vi "Delete last element.vi"(8 "error in":errorcluster, 11 "Path in":string) -> (0 "error out":errorcluster, 2 "Path Array Out":string[](array[string]), 3 "Element Array Out":string[](array[string]))   [LabVIEW 2015]
uses:
  <vilib>/regexp/Match Regular Expression.xnode
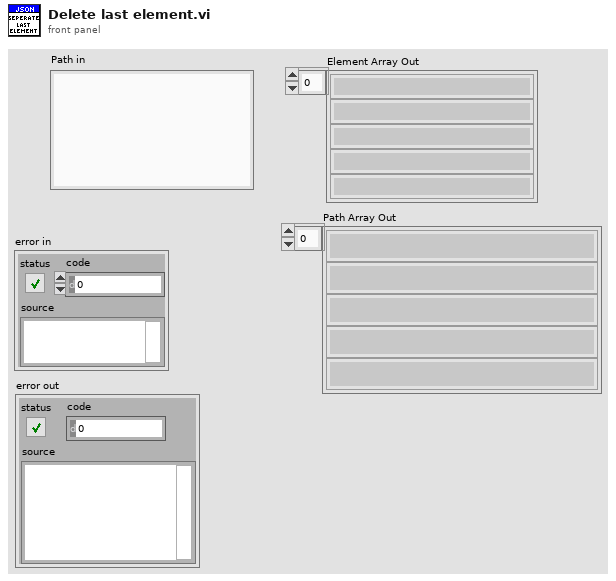
[diagram p1: front panel]
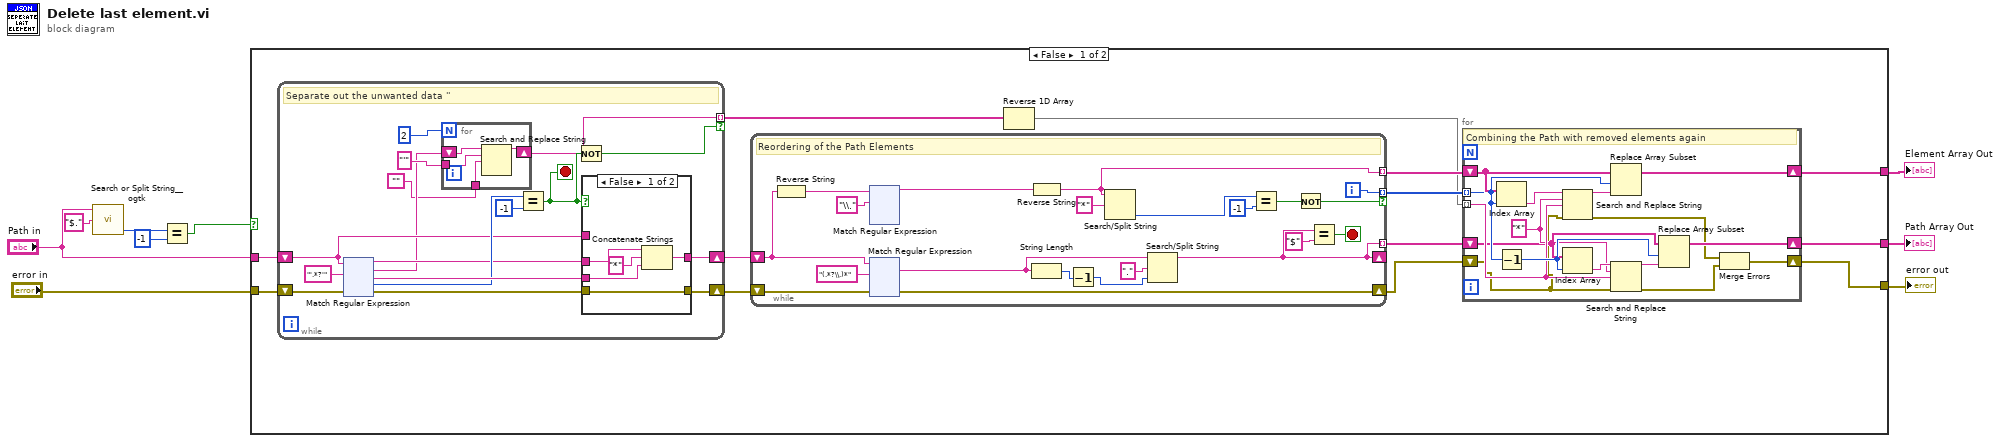
[diagram p0: block diagram]
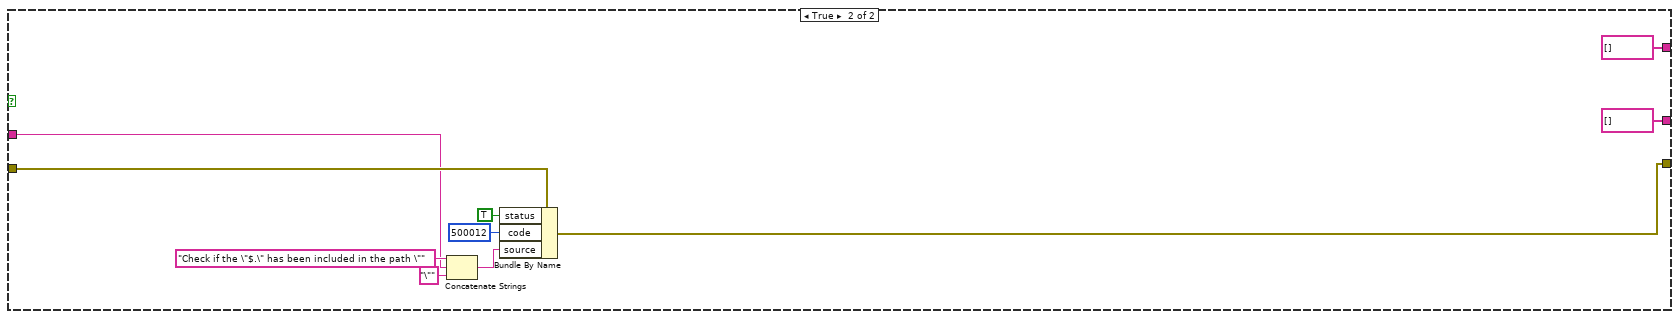
[diagram p3: hidden frame]
diagram:
  n1 = call <userlib>:"Search or Split String__ogtk.vi"("search string/char (-)"="$.", "string"="Path in") -> ("offset after match"=w3:i32)  [unwired: 1 in, 2 out]
  n2 = Equal?(x=w3, y=-1) -> (x = y?=w1:bool)
  n3 = case shown="False" w1 {
    tunnel: [w18 string[] []] -> w9
    tunnel: [w17 string[] []] -> w8
    tunnel: "error in" -> [w16 w439]
    tunnel: [w13 w432] -> w6
    tunnel: "Path in" -> [w10 w435]
    frame False {
      n4 = while {
        shift-right: [w302] -> w22
        shift-left: w10 -> [w298]
        tunnel: [w289] -> w12 mode=indexing if=w297
        shift-right: [w294] -> w15
        shift-left: w16 -> [w296]
        stop <- w299 stop-if-true
        # "Separate out the unwanted data ''"
        n5 = xnode "Match Regular Expression"("input string"=w298, "regular expression"="'.*?'", "error in"=w296) -> ("before match"=w300:string, "whole match"=w290:string, "after match"=w303:string, "offset past match"=w301:i32, "error out"=w295:errorcluster)  [unwired: 3 in]
        n6 = for {
          N: 2 -> [_]
          tunnel: "'" ("substring (\"\")") -> [w306]
          shift-right: [w307] -> w289
          shift-left: w290 -> [w308]
          tunnel: "" -> [w305]
          n7 = Search and Replace String(input string=w308, search string=w306, replace string=w305) -> (result string=w307:string)  [unwired: 5 in, 3 out]
        }
        n8 = Equal?(x=w301, y=-1) -> (x = y?=w299:bool)
        n9 = Not(x=w299) -> (.not. x?=w297:bool)
        n10 = case shown="False" w299 {
          tunnel: w303 -> [w313 _]
          tunnel: [w312 w315] -> w302
          tunnel: w300 -> [w311 _]
          tunnel: w298 -> [_ w315]
          tunnel: w295 -> [w309 w314]
          tunnel: [w309 w314] -> w294
          frame False {
            n11 = Concatenate Strings(w311, "*" ("string"), w313) -> (w312:string)
          }
          frame True {
          }
        }
      }
      n12 = while {
        shift-right: [w47] -> w14
        shift-left: w15 -> [w49]
        tunnel: [w44] -> w21 mode=indexing
        shift-right: [w46] -> _
        shift-left: w22 -> [w52]
        tunnel: [w46] -> w20 mode=indexing
        tunnel: [w41] -> w19 mode=indexing if=w39
        i -> [w41]
        stop <- w50 stop-if-true
        # "Reordering of the Path Elements"
        n13 = Reverse String(1:w52) -> (0:w55:string)
        n14 = xnode "Match Regular Expression"("input string"=w55, "regular expression"="\\.") -> ("before match"=w53:string)  [unwired: 4 in, 4 out]
        n15 = xnode "Match Regular Expression"("input string"=w52, "regular expression"="(.*?\\.)*", "error in"=w49) -> ("whole match"=w48:string, "error out"=w47:errorcluster)  [unwired: 3 in, 3 out]
        n16 = Reverse String(1:w53) -> (0:w44:string)
        n17 = String Length(string=w48) -> (length=w57:i32)
        n18 = Decrement(x=w57) -> (x-1=w56:i32)
        n19 = Search/Split String(string=w44, search string/char (-)="*") -> (offset of match=w43:i32)  [unwired: 1 in, 2 out]
        n20 = Search/Split String(string=w48, search string/char (-)=".", offset (0)=w56) -> (substring before match=w46:string)  [unwired: 2 out]
        n21 = Equal?(x=w43, y=-1) -> (x = y?=w40:bool)
        n22 = Not(x=w40) -> (.not. x?=w39:bool)
        n23 = Equal?(x=w46, y="$") -> (x = y?=w50:bool)
      }
      n24 = Reverse 1D Array(array=w12) -> (reversed array=w11:string[])
      n25 = for {
        tunnel: w19 -> [w37] mode=indexing
        tunnel: w11 -> [w29] mode=indexing
        shift-right: [w36] -> w18
        shift-left: w21 -> [w38]
        shift-right: [w32] -> w17
        shift-left: w20 -> [w27]
        shift-right: [w23] -> w13
        shift-left: w14 -> [w26]
        w28 = "*" ("search string")
        # "Combining the Path with removed elements again"
        n26 = Index Array(array=w38, index=w37) -> (element=w31:string)
        n27 = Decrement(x=w37) -> (x-1=w35:i32)
        n28 = Search and Replace String(input string=w31, search string=w28, replace string=w29, error in=w26) -> (result string=w30:string, error out=w25:errorcluster)  [unwired: 4 in, 2 out]
        n29 = Index Array(array=w27, index=w35) -> (element=w34:string)
        n30 = Replace Array Subset(array=w38, new element=w30, index=w37) -> (w36:string[])
        n31 = Search and Replace String(input string=w34, search string=w28, replace string=w29, error in=w26) -> (result string=w33:string, error out=w24:errorcluster)  [unwired: 4 in, 2 out]
        n32 = Replace Array Subset(array=w27, new element=w33, index=w35) -> (w32:string[])
        n33 = Merge Errors(w25, w24) -> (w23:errorcluster)
      }
    }
    frame True {
      n34 = Concatenate Strings("Check if the \"$.\" has been included in the path \"" ("source"), w435, "\"" ("string")) -> (w433:string)
      n35 = Bundle By Name(cluster=w439, "status"=TRUE, "code"=500012, "source"=w433) -> (w432:errorcluster)
    }
  }
  "error out" <- w6
  "Element Array Out" <- w9
  "Path Array Out" <- w8
